vi "CRYChange Autosave Flatten Data by One.vi"(7 "Option":string, 11 "Flatten Autosave In":string) -> (3 "Flatten Autosave Out":string)   [LabVIEW 2013]
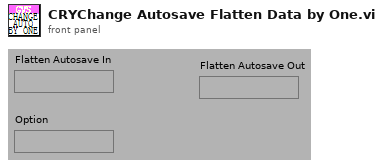
[diagram p1: front panel]
types:
  T1 = typedef "CRYAuto Save Cluster.ctl" = cluster{"Name":string, "save":enum16{"Data", "Results", "Waveforms"}, "Item Names":string[], "Autosave folder":path, "data format":u16, "filename option":enum16{"auto", "prompt"}, "fn construction":i32[], "layout":enum16{"rows", "columns"}, "notation":enum16{"sci", "float"}, "precision":i32, "prompt comment":bool, "header":enum16{"none", "standard", "custom"}, "custom header":string, "serial no.":bool, "User defined":string, "delimiter":enum16{"tab", "comma", "space", "other"}, "other delim":string, "axes":cluster{"x":bool, "y":bool, "z":bool}, "Time Stamp":bool, "Lot No.":bool, "Operator":bool, "Excel Template":string, "New or Append":u16, "Data":u16, "Help":string, "Tab Value":enum32{"Setting", "Help"}, "UDL or DSN":path, "User Default":bool, "Selector":i32, "Axis":u16, "Value Name":string, "format string":cluster{"dB Format String out":string, "Lin Format String out":string}, "DBPath":path}
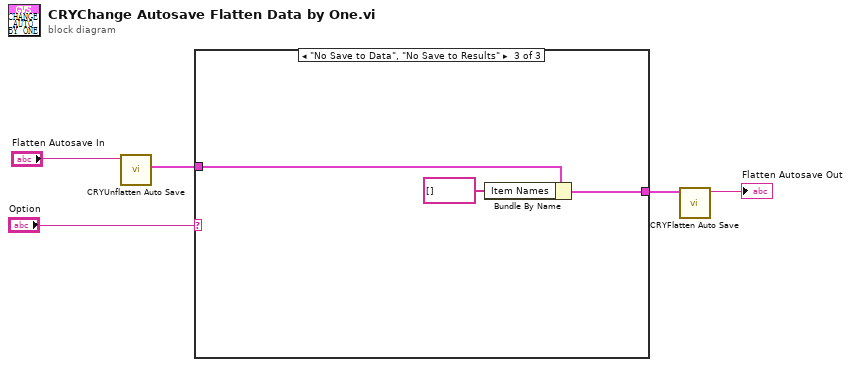
[diagram p0: block diagram]
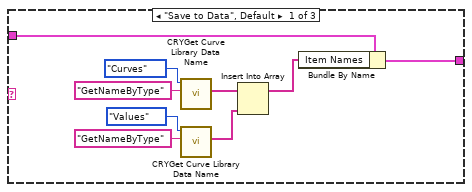
[diagram p2: hidden frame]
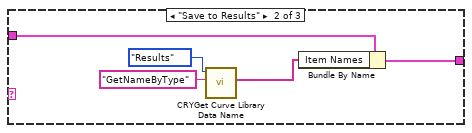
[diagram p3: hidden frame]
diagram:
  n1 = call "CRYUnflatten Auto Save.vi"("Flatten Auto Save"="Flatten Autosave In") -> ("Auto save"=w3:T1)  [unwired: 8 in, 2 out]
  n2 = case shown="\"No Save to Data\", \"No Save to Results\"" "Option" {
    tunnel: w3 -> [w14 w19 w22]
    tunnel: [w6 w16 w21] -> w1
    frame "Save to Data", Default {
      n3 = call "CRYGet Curve Library Data Name.vi"("sAction"="GetNameByType", "Type"=enum16{"Curves", "Values", "Results", "WFM"}."Curves") -> ("sNames"=w9:string[])  [unwired: 6 in, 3 out]
      n4 = call "CRYGet Curve Library Data Name.vi"("sAction"="GetNameByType", "Type"=enum16{"Curves", "Values", "Results", "WFM"}."Values") -> ("sNames"=w8:string[])  [unwired: 6 in, 3 out]
      n5 = Insert Into Array(array=w9, new element=w8) -> (w7:string[])  [unwired: 1 in]
      n6 = Bundle By Name(cluster=w14, "Item Names"=w7) -> (w6:T1)
    }
    frame "Save to Results" {
      n7 = call "CRYGet Curve Library Data Name.vi"("sAction"="GetNameByType", "Type"=enum16{"Curves", "Values", "Results", "WFM"}."Results") -> ("sNames"=w15:string[])  [unwired: 6 in, 3 out]
      n8 = Bundle By Name(cluster=w19, "Item Names"=w15) -> (w16:T1)
    }
    frame "No Save to Data", "No Save to Results" {
      n9 = Bundle By Name(cluster=w22, "Item Names"=string[] []) -> (w21:T1)
    }
  }
  n10 = call "CRYFlatten Auto Save.vi"("Auto Save"=w1) -> ("Auto Save flattened"=→"Flatten Autosave Out":string)  [unwired: 10 in]
